vi "NOx parse.vi"(1 "NOx Input array":dbl[](array[numeric])=[0.0, 0.0, 0.0, 0.0]) -> (0 "NOx output array":dbl[](array[numeric]))   [LabVIEW 2011]
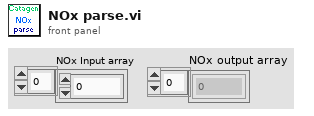
[diagram p1: front panel]
types:
  T1 = cluster{"NOx (bits)":i16, "O2 (bits)":u16, "Sensor Supply Status":u8, "Sensor Temperature Status":u8, "NOx Signal Status":u8, "O2 Signal Status":u8, "Heater Mode Status":u8, "Heater Circuit Status":u8, "NOx Circuit Status":u8, "O2 Circuit Status":u8, "NOx Sensor Module Present":bool}
  T2 = cluster{"NOx (ppm)":i16, "O2 (%)":sgl, "Sensor Supply Status":u8, "Sensor Temperature Status":u8, "NOx Signal Status":u8, "O2 Signal Status":u8, "Heater Mode Status":u8, "Heater Circuit Status":u8, "NOx Circuit Status":u8, "O2 Circuit Status":u8, "NOx Sensor Module Present":bool}
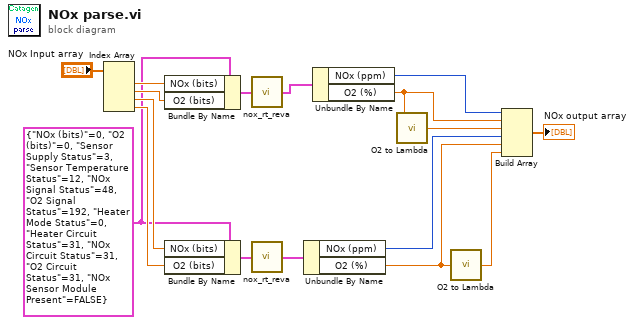
[diagram p0: block diagram]
diagram:
  w8 = T1 {"NOx (bits)"=0, "O2 (bits)"=0, "Sensor Supply Status"=3, "Sensor Temperature Status"=12, "NOx Signal Status"=48, "O2 Signal Status"=192, "Heater Mode Status"=0, "Heater Circuit Status"=31, "NOx Circuit Status"=31, "O2 Circuit Status"=31, "NOx Sensor Module Present"=FALSE} ("NOxSensorData 1")
  n1 = Index Array(array="NOx Input array") -> (element #1=w13:dbl, element #2=w11:dbl, element #3=w10:dbl, element #4=w9:dbl)  [unwired: 4 in]
  n2 = Bundle By Name(cluster=w8, "NOx (bits)"=w13, "O2 (bits)"=w11) -> (w16:T1)
  n3 = Bundle By Name(cluster=w8, "NOx (bits)"=w10, "O2 (bits)"=w9) -> (w15:T1)
  n4 = call <vilib>:"nox_rt_reva.vi"("NOxSensorDataFromFPGA"=w16) -> ("NOxSensorData"=w17:T2)
  n5 = call <vilib>:"nox_rt_reva.vi"("NOxSensorDataFromFPGA"=w15) -> ("NOxSensorData"=w14:T2)
  n6 = Unbundle By Name(w14) -> ("NOx (ppm)"=w4:i16, "O2 (%)"=w3:sgl)
  n7 = Unbundle By Name(w17) -> ("NOx (ppm)"=w7:i16, "O2 (%)"=w6:sgl)
  n8 = call "O2 to Lambda.vi"("O2 %"=w6) -> ("Lambda"=w5:dbl)
  n9 = call "O2 to Lambda.vi"("O2 %"=w3) -> ("Lambda"=w2:dbl)
  n10 = Build Array(w7, w6, w5, w4, w3, w2) -> (→"NOx output array":dbl[])
